vi "display_data Message_Init.vi"(8 "error in (no error)":errorcluster, 11 "object in":refnum<class "display_data Message.lvclass">) -> (0 "error out":errorcluster, 3 "object out":refnum<class "display_data Message.lvclass">)   [LabVIEW 2018, in "ClientMessaging.lvlib" / "display_data Message.lvclass"]
uses:
  display_data Message.lvclass
  C:/Users/gavin/Documents/Programming/LabVIEW/JuPyterClient/Base Classes/Message Class/Message Class.lvclass
  display_data Message.lvclass/display_data Message.ctl
  Base Classes/Message Class/Message Class.lvclass
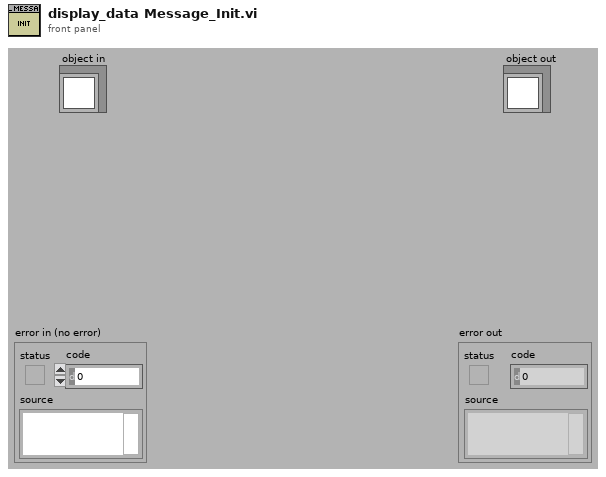
[diagram p1: front panel]
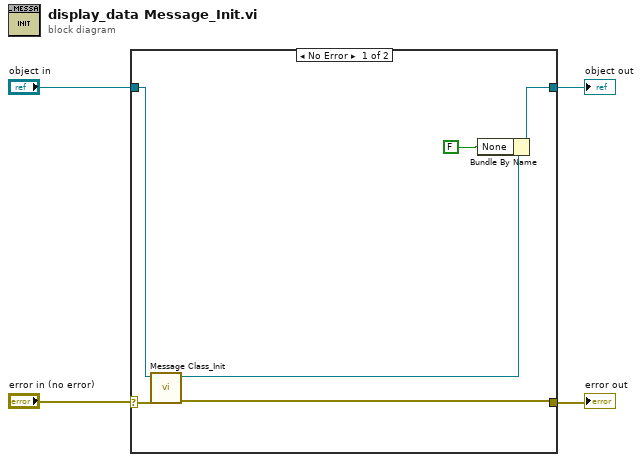
[diagram p0: block diagram]
diagram:
  n1 = case shown="No Error" "error in (no error)" {
    selector: "error in (no error)" -> [w7 w11]
    tunnel: "object in" -> [w8 w12]
    tunnel: [w10 w12] -> w3
    tunnel: [w5 w11] -> w1
    frame No Error {
      n2 = call "Message Class_Init.vi"("error in (no error)"=w7, "object in"=w8) -> ("error out"=w5:errorcluster, "object out"=w6:refnum<class "display_data Message.lvclass">)  [unwired: 8 in]
      n3 = Bundle By Name(cluster=w6, "None"=FALSE) -> (w10:refnum<class "display_data Message.lvclass">)
    }
    frame Error {
    }
  }
  "object out" <- w3
  "error out" <- w1
